vi "SysConfig.vi"() -> (1 "SysConfigCluster":T3)   [LabVIEW 2020]
uses:
  <vilib>/addons/_JKI.lib/Serialization/JSON/JKI JSON Serialization.lvlib
  <userlib>/_OpenG.lib/file/file.llb/openg_file.lvlib
  <instrlib>/niScope/Controls/niScope trigger source.ctl
  FLImDAQ.ctl
panel:
  in  "FLImDAQ":T1={"Digitizer 1"="", "Digitizer 2"="", "Channel"=enum."Channel 0&1", "trigger source"="VAL_EXTERNAL", "trigger level"=1.0, "trigger delay"=2e-08, "min sample rate"=2500000000.0, "min record length"=300, "vertical range"=2.0, "vertical offset"=0.7, "Waveform to Avg"=10000000} caption="FLIm DAQ Configuration" {"trigger delay" format="%^#.4e"; "trigger level" format="%.4f"; "vertical offset" format="%.4f"; "vertical range" format="%.2f"; "min record length" format="%^#.4e"; "min sample rate" min=0.0 max=3.5 step=0.5 format="%.2f"}
  in  "LoadDefault":bool
  in  "AimingBeamEnable?":bool=TRUE
  in  "Cancel":bool
  in  "Confirm":bool
  in  "Ch3AutoGain?":bool=TRUE
  in  "Ch2AutoGain?":bool=TRUE
  in  "Ch1AutoGain?":bool=TRUE
  in  "Ch3Enable?":bool=TRUE
  in  "Ch2Enable?":bool=TRUE
  in  "Ch1Enable?":bool=TRUE
  # "System Configuration"
  # "Channel 1:"
  # "Channel 2:"
  # "Channel 3:"
  # "Aimging Beam:"
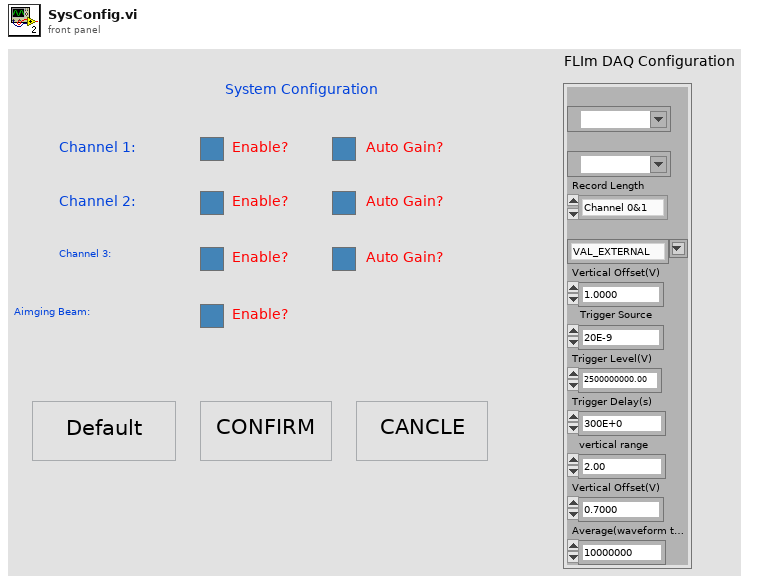
[diagram p1: front panel]
types:
  T1 = typedef "FLImDAQ.ctl" = cluster{"Digitizer 1":refnum<k15>, "Digitizer 2":refnum<k15>, "Channel":enum16{"Channel 0", "Channel 1", "Channel 0&1"}, "trigger source":T2, "trigger level":dbl, "trigger delay":dbl, "min sample rate":dbl, "min record length":i32, "vertical range":dbl, "vertical offset":dbl, "Waveform to Avg":i32}
  T2 = typedef "niScope trigger source.ctl" = string
  T3 = cluster{"Ch1Enable?":bool, "Ch2Enable?":bool, "Ch3Enable?":bool, "Ch1AutoGain?":bool, "Ch2AutoGain?":bool, "Ch3AutoGain?":bool, "AimingBeamEnable?":bool}
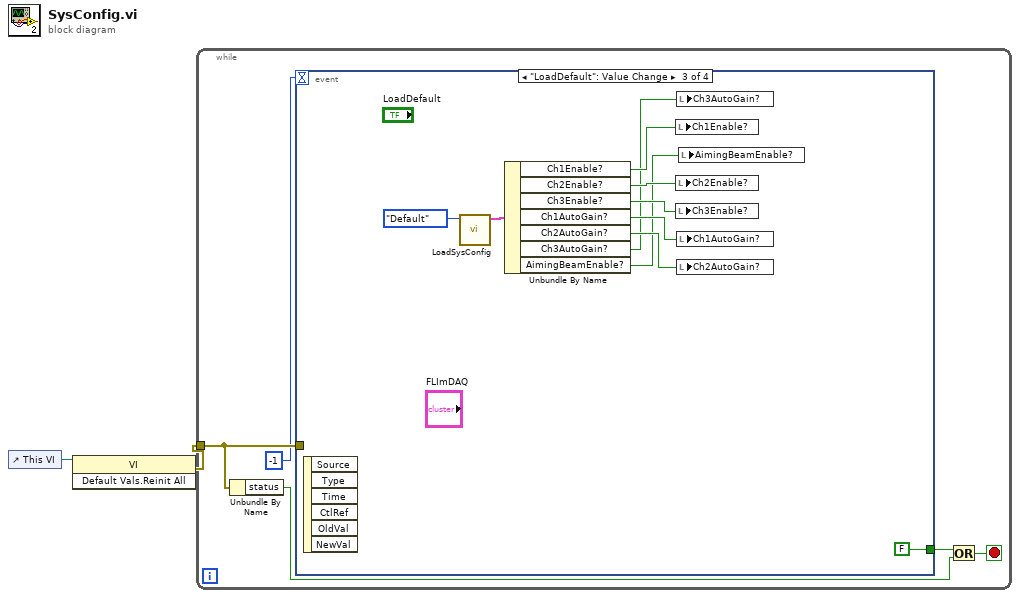
[diagram p0: block diagram]
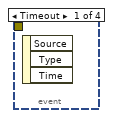
[diagram p2: hidden frame]
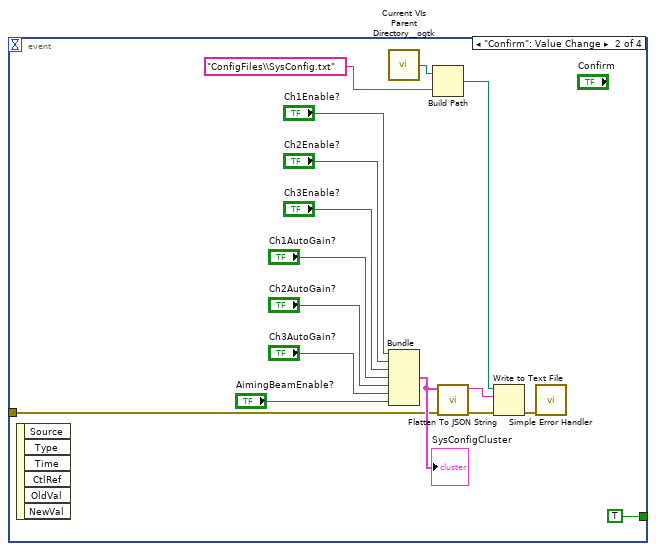
[diagram p3: hidden frame]
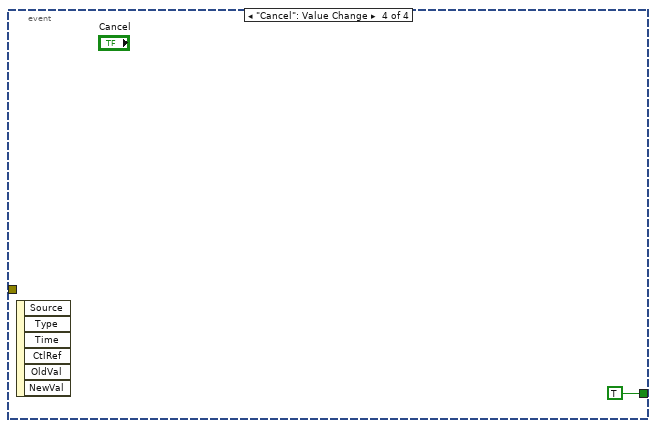
[diagram p4: hidden frame]
diagram:
  n1 = control-ref of="This VI"() -> (w2:refnum<vi>)
  n2 = invoke class="VI" method="Default Vals.Reinit All"(reference=w2) -> (error out=w1:errorcluster)  [unwired: 2 in, 2 out]
  n3 = while {
    tunnel: w1 -> [w7]
    stop <- w4 stop-if-true
    n4 = Unbundle By Name(w7) -> ("status"=w5:bool)
    n5 = event shown="[2] \"LoadDefault\": Value Change" {
      selector: _ -> [_ _ _ _]
      dyn-events: _ -> [_ _ _ _]
      timeout: -1 -> [_ _ _ _]
      tunnel: [_ TRUE FALSE TRUE] -> w6
      tunnel: w7 -> [_ w14 _ _]
      event Timeout {
        n6 = event-data() -> ()  [unwired: 1 in, 3 out]
      }
      event "Confirm": Value Change {
        n7 = event-data() -> ()  [unwired: 1 in, 6 out]
        n8 = call <userlib>:"Current VIs Parent Directory__ogtk.vi"() -> ("Parent Directory (+ Relative)"=w11:path)  [unwired: 5 in]
        n9 = Bundle("Ch1Enable?"="Ch1Enable?", "Ch2Enable?"="Ch2Enable?", "Ch3Enable?"="Ch3Enable?", "Ch1AutoGain?"="Ch1AutoGain?", "Ch2AutoGain?"="Ch2AutoGain?", "Ch3AutoGain?"="Ch3AutoGain?", "AimingBeamEnable?"="AimingBeamEnable?") -> (w15:T3)  [unwired: 1 in]
        "SysConfigCluster" <- w15
        n10 = Build Path(base path=w11, name or relative path="ConfigFiles\\SysConfig.txt") -> (appended path=w9:path)
        n11 = call <vilib>:"Flatten To JSON String.vi"("error in"=w14, "Variant"=w15) -> ("error out"=w12:errorcluster, "JSON String"=w13:string)  [unwired: 8 in]
        n12 = Write to Text File(file (use dialog)=w9, text=w13, error in=w12) -> (error out=w8:errorcluster)  [unwired: 1 in, 2 out]
        n13 = call <vilib>:"Simple Error Handler.vi"("error in (no error)"=w8) -> ()  [unwired: 4 in, 5 out]
      }
      event "LoadDefault": Value Change {
        n14 = event-data() -> ()  [unwired: 1 in, 6 out]
        n15 = call "LoadSysConfig.vi"("Enum"=enum16{"LastUse", "Default"}."Default") -> ("SysConfigCluster"=w32:T3)  [unwired: 9 in, 1 out]
        n16 = Unbundle By Name(w32) -> ("Ch1Enable?"=w30:bool, "Ch2Enable?"=w29:bool, "Ch3Enable?"=w28:bool, "Ch1AutoGain?"=w27:bool, "Ch2AutoGain?"=w26:bool, "Ch3AutoGain?"=w25:bool, "AimingBeamEnable?"=w24:bool)
        n17 = local write "Ch1Enable?"(w30) -> ()
        n18 = local write "Ch2Enable?"(w29) -> ()
        n19 = local write "Ch3Enable?"(w28) -> ()
        n20 = local write "Ch3AutoGain?"(w25) -> ()
        n21 = local write "Ch1AutoGain?"(w27) -> ()
        n22 = local write "Ch2AutoGain?"(w26) -> ()
        n23 = local write "AimingBeamEnable?"(w24) -> ()
      }
      event "Cancel": Value Change {
        n24 = event-data() -> ()  [unwired: 1 in, 6 out]
      }
    }
    n25 = Or(x=w6, y=w5) -> (x .or. y?=w4:bool)
  }
